vi "aggregator - pid.vi"(0 "df":dbl=100.0, 1 "low":dbl=1.0, 2 "threshold":dbl=1.0, 3 "dz":dbl=-9.0, 4 "dz0":dbl=-6.0, 5 "high":dbl=1.0, 6 "requested size":i32=10, 7 "P":dbl=0.1, 8 "negative":i32=2, 10 "first time":bool, 11 "I":dbl=1.0, 12 "requested averaging interval":i32=9, 13 "D":dbl=1.0) -> (14 "new df":dbl, 17 "above ?":bool, 18 "thershold ?":bool, 19 "heater":dbl)   [LabVIEW 2012]
panel:
  out "mean":dbl
  out "slope":dbl
  out "interpolated average":dbl
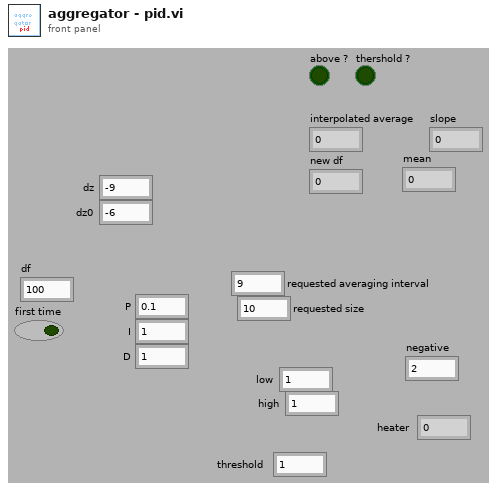
[diagram p1: front panel]
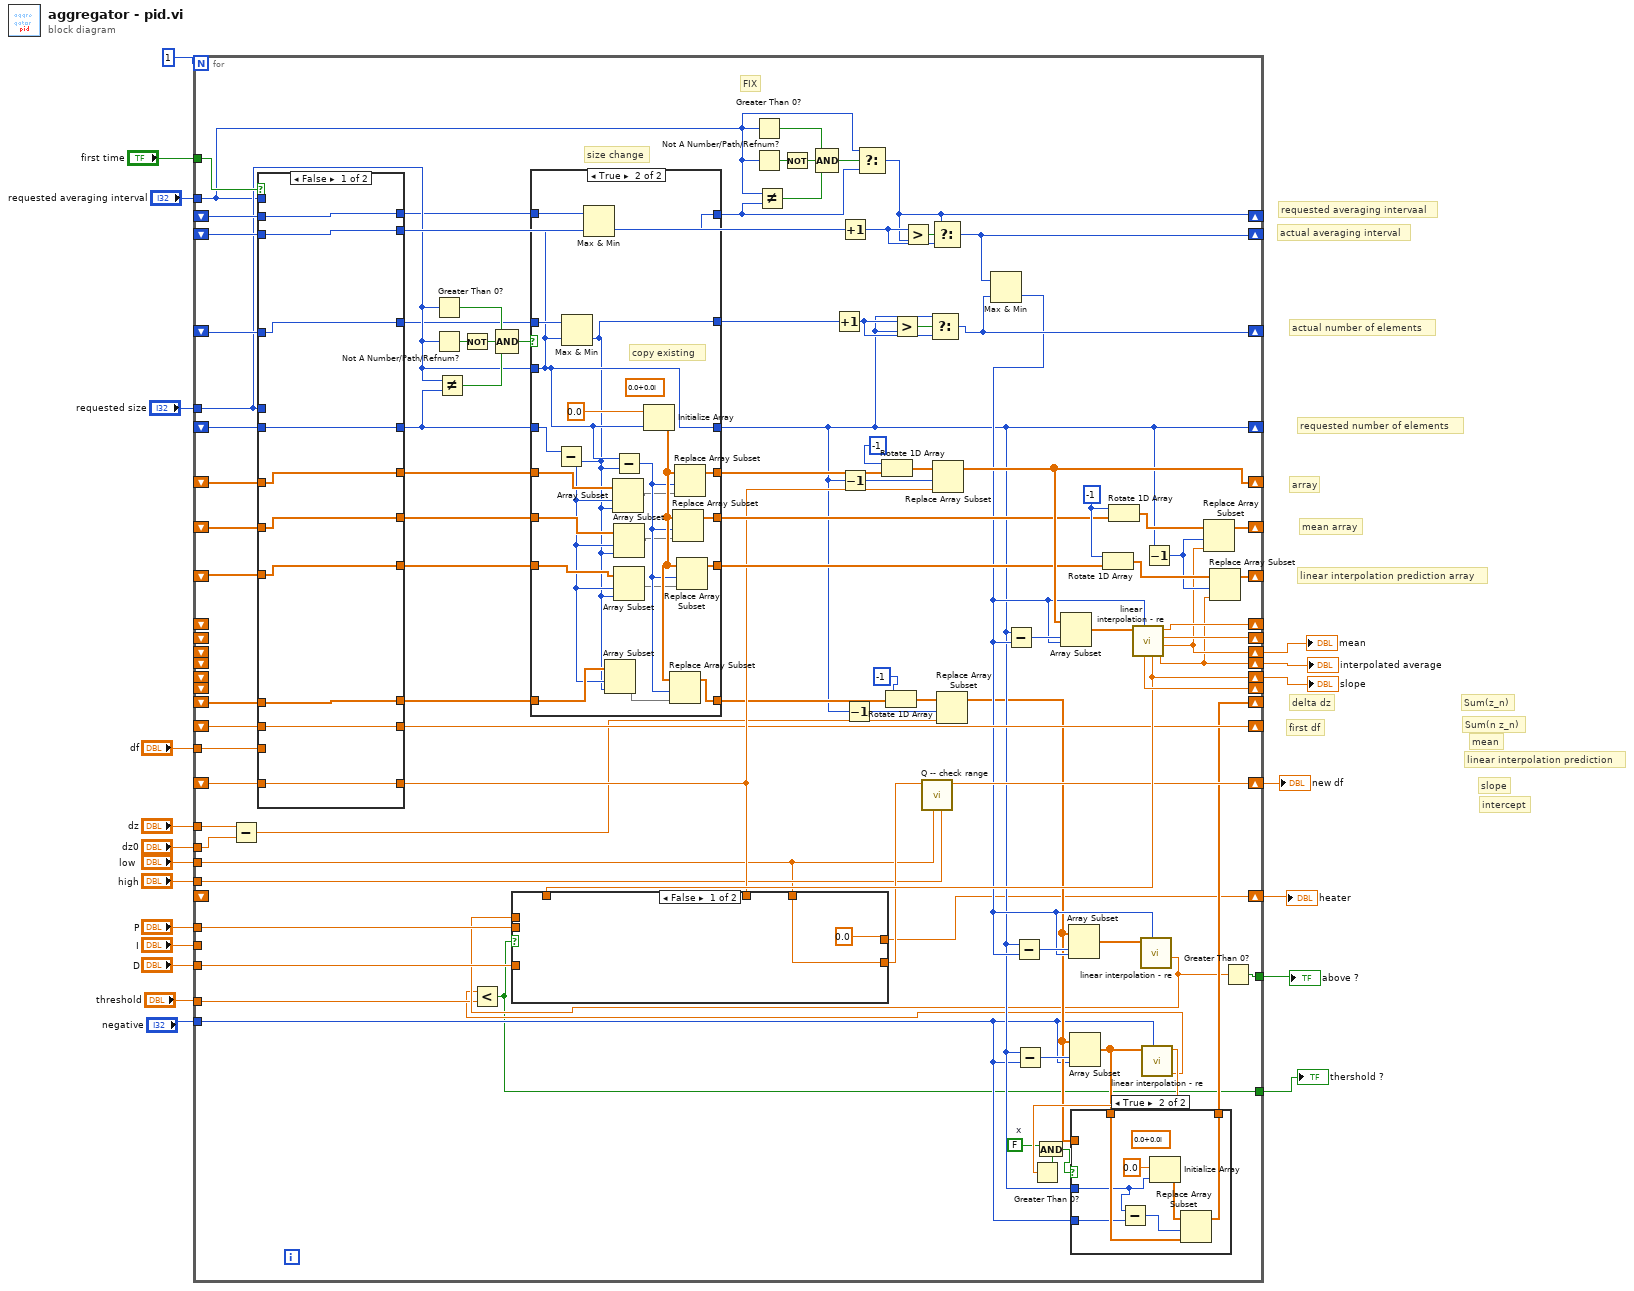
[diagram p0: block diagram]
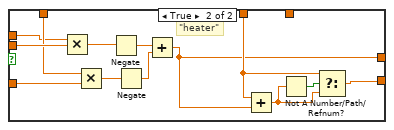
[diagram p2: hidden frame]
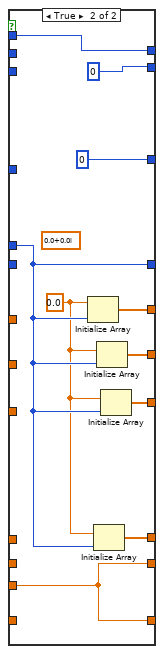
[diagram p5: hidden frame]
diagram:
  # "delta dz"
  # "first df"
  # "array"
  # "actual averaging interval"
  # "requested averaging intervaal"
  # "linear interpolation prediction"
  # "mean"
  # "intercept"
  # "slope"
  # "linear interpolation prediction array"
  # "mean array"
  # "Sum(n z_n)"
  # "Sum(z_n)"
  # "requested number of elements"
  # "actual number of elements"
  n1 = for {
    N: 1 -> [_]
    tunnel: "first time" -> [w94]
    shift-right: [w64] -> _
    shift-left: _ -> [w117]
    tunnel: "requested size" -> [w81]
    tunnel: "df" -> [w52]
    shift-right: [w96] -> _
    shift-left: _ -> [w114]
    shift-right: [w36] -> _
    shift-left: _ -> [w110]
    shift-right: [w103] -> _
    shift-left: _ -> [w109]
    shift-right: [w102] -> _
    shift-left: _ -> [w108]
    shift-right: [w92] -> _
    shift-left: _ -> [_]
    shift-right: [w91] -> _
    shift-left: _ -> [_]
    shift-right: [w57] -> w15
    shift-left: _ -> [_]
    shift-right: [w58] -> _
    shift-left: _ -> [_]
    shift-right: [w90] -> w14
    shift-left: _ -> [_]
    shift-right: [w89] -> w16
    shift-left: _ -> [_]
    shift-right: [w63] -> _
    shift-left: _ -> [w98]
    shift-right: [w65] -> _
    shift-left: _ -> [w97]
    tunnel: "requested averaging interval" -> [w67]
    tunnel: "P" -> [w62]
    tunnel: "dz" -> [w61]
    tunnel: "dz0" -> [w60]
    tunnel: "D" -> [w59]
    tunnel: "I" -> [_]
    shift-right: [w53] -> w8
    shift-left: _ -> [w55]
    shift-right: [w50] -> _
    shift-left: _ -> [w51]
    tunnel: "low" -> [w29]
    tunnel: "high" -> [w49]
    tunnel: [w48] -> w5
    shift-right: [w34] -> _
    shift-left: _ -> [w46]
    tunnel: "negative" -> [w32]
    shift-right: [w31] -> w3
    shift-left: _ -> [_]
    tunnel: "threshold" -> [w28]
    tunnel: [w22] -> w1
    w25 = FALSE  # x
    w105 = -1 ("n")
    # "FIX"
    # "size change"
    n2 = Subtract(x=w61, y=w60) -> (x-y=w24:dbl)
    n3 = case shown="False" w94 {
      tunnel: w117 -> [w178 _]
      tunnel: [w178 0] -> w79
      tunnel: w114 -> [w175 _]
      tunnel: w81 -> [_ w182]
      tunnel: w110 -> [w176 _]
      tunnel: w109 -> [w174 _]
      tunnel: w108 -> [w173 _]
      tunnel: [w175 w186] -> w83
      tunnel: [w174 w185] -> w76
      tunnel: [w173 w184] -> w77
      tunnel: [w179 0] -> w100
      tunnel: w98 -> [w179 _]
      tunnel: w67 -> [_ w187]
      tunnel: w97 -> [w177 _]
      tunnel: [w177 w187] -> w73
      tunnel: [w176 w182] -> w80
      tunnel: [w172 w183] -> w56
      tunnel: w52 -> [_ w183]
      tunnel: w55 -> [w172 _]
      tunnel: [w171 w183] -> w50
      tunnel: w51 -> [w171 _]
      tunnel: [w170 w180] -> w47
      tunnel: w46 -> [w170 _]
      frame False {
      }
      frame True {
        w181 = 0.0
        (unwired) cdb 0.0+0.0i
        n4 = Initialize Array(w181, w182) -> (w186:dbl[])
        n5 = Initialize Array(w181, w182) -> (w180:dbl[])
        n6 = Initialize Array(w181, w182) -> (w185:dbl[])
        n7 = Initialize Array(w181, w182) -> (w184:dbl[])
      }
    }
    n8 = Greater Than 0?(x=w81) -> (x > 0?=w87:bool)
    n9 = Not A Number/Path/Refnum?(number/path/refnum=w81) -> (NaN/Path/Refnum?=w88:bool)
    n10 = Not Equal?(x=w81, y=w80) -> (x != y?=w85:bool)
    n11 = Not(x=w88) -> (.not. x?=w86:bool)
    n12 = Compound Arithmetic op=AND(w87, w86, w85) -> (w84:bool)
    n13 = case shown="True" w84 {
      tunnel: [w147 w148] -> w78
      tunnel: w79 -> [w147 w169]
      tunnel: [w146 w163] -> w36
      tunnel: w80 -> [w146 w150]
      tunnel: [w145 w168] -> w82
      tunnel: w83 -> [w145 w154]
      tunnel: w81 -> [_ w163]
      tunnel: w77 -> [w143 w158]
      tunnel: w76 -> [w144 w156]
      tunnel: [w144 w167] -> w75
      tunnel: [w143 w166] -> w74
      tunnel: w73 -> [w142 w165]
      tunnel: [w142 w164] -> w66
      tunnel: w47 -> [w141 w152]
      tunnel: [w141 w159] -> w43
      frame False {
      }
      frame True {
        (unwired) cdb 0.0+0.0i
        # "copy existing"
        n14 = Max & Min(x=w169, y=w163) -> (min(x,y)=w148:i32)  [unwired: 1 out]
        n15 = Subtract(x=w150, y=w148) -> (x-y=w149:i32)
        n16 = Max & Min(x=w165, y=w163) -> (min(x,y)=w164:i32)  [unwired: 1 out]
        n17 = Array Subset(array=w152, index=w149, length=w148) -> (w151:dbl[])
        n18 = Array Subset(array=w154, index=w149, length=w148) -> (w153:dbl[])
        n19 = Subtract(x=w163, y=w148) -> (x-y=w160:i32)
        n20 = Array Subset(array=w156, index=w149, length=w148) -> (w155:dbl[])
        n21 = Array Subset(array=w158, index=w149, length=w148) -> (w157:dbl[])
        n22 = Initialize Array(0.0, w163) -> (w161:dbl[])
        n23 = Replace Array Subset(array=w161, new element=w151, index=w160) -> (w159:dbl[])
        n24 = Replace Array Subset(array=w161, new element=w155, index=w160) -> (w167:dbl[])
        n25 = Replace Array Subset(array=w161, new element=w153, index=w160) -> (w168:dbl[])
        n26 = Replace Array Subset(array=w161, new element=w157, index=w160) -> (w166:dbl[])
      }
    }
    n27 = Greater Than 0?(x=w67) -> (x > 0?=w71:bool)
    n28 = Not A Number/Path/Refnum?(number/path/refnum=w67) -> (NaN/Path/Refnum?=w72:bool)
    n29 = Not Equal?(x=w67, y=w66) -> (x != y?=w69:bool)
    n30 = Not(x=w72) -> (.not. x?=w70:bool)
    n31 = Compound Arithmetic op=AND(w71, w70, w69) -> (w68:bool)
    n32 = Increment(x=w78) -> (x+1=w115:i32)
    n33 = Increment(x=w100) -> (x+1=w99:i32)
    n34 = Decrement(x=w36) -> (x-1=w112:i32)
    n35 = Decrement(x=w36) -> (x-1=w45:i32)
    n36 = Select(t=w67, s=w68, f=w66) -> (s? t:f=w65:i32)
    n37 = Rotate 1D Array(1:w82, 2:-1 ("n")) -> (0:w111:dbl[])
    n38 = Rotate 1D Array(1:w43, 2:-1 ("n")) -> (0:w44:dbl[])
    n39 = Greater?(x=w115, y=w36) -> (0:w116:bool)
    n40 = Greater?(x=w99, y=w65) -> (0:w101:bool)
    n41 = Select(t=w36, s=w116, f=w115) -> (s? t:f=w64:i32)
    n42 = Select(t=w65, s=w101, f=w99) -> (s? t:f=w63:i32)
    n43 = Replace Array Subset(array=w111, new element=w56, index=w112) -> (w96:dbl[])
    n44 = Replace Array Subset(array=w44, new element=w24, index=w45) -> (w33:dbl[])
    n45 = Max & Min(x=w63, y=w64) -> (min(x,y)=w39:i32)  [unwired: 1 out]
    n46 = Subtract(x=w36, y=w39) -> (x-y=w95:i32)
    n47 = Subtract(x=w36, y=w39) -> (x-y=w41:i32)
    n48 = Subtract(x=w36, y=w32) -> (x-y=w38:i32)
    n49 = Array Subset(array=w96, index=w95, length=w39) -> (w93:dbl[])
    n50 = Array Subset(array=w33, index=w41, length=w39) -> (w40:dbl[])
    n51 = Array Subset(array=w33, index=w38, length=w32) -> (w35:dbl[])
    n52 = Rotate 1D Array(1:w74, 2:w105) -> (0:w106:dbl[])
    n53 = Rotate 1D Array(1:w75, 2:w105) -> (0:w107:dbl[])
    n54 = call "linear interpolation - re.vi"("n"=w39, "Array"=w93) -> ("interpolated average"=w89:dbl, "mean"=w90:dbl, "sum n z_n"=w91:dbl, "sum z_n"=w92:dbl, "slope"=w57:dbl, "intercept"=w58:dbl)  [unwired: 4 in]
    n55 = call "linear interpolation - re.vi"("n"=w39, "Array"=w40) -> ("mean"=w30:dbl)  [unwired: 4 in, 5 out]
    n56 = call "linear interpolation - re.vi"("n"=w32, "Array"=w35) -> ("interpolated average"=w23:dbl, "sum z_n"=w37:dbl)  [unwired: 4 in, 4 out]
    n57 = Less?(x=w23, y=w28) -> (x < y?=w22:bool)
    n58 = case shown="False" w22 {
      tunnel: w62 -> [_ w132]
      tunnel: w59 -> [_ w131]
      tunnel: w57 -> [_ w126]
      tunnel: w56 -> [_ w123]
      tunnel: [w119 w122] -> w54
      tunnel: [0.0 w121] -> w31
      tunnel: w30 -> [_ w120]
      tunnel: w29 -> [w119 _]
      frame False {
      }
      frame True {
        # "\"heater\""
        n59 = Multiply(x=w120, y=w132) -> (x*y=w130:dbl)
        n60 = Multiply(x=w126, y=w131) -> (x*y=w129:dbl)
        n61 = Negate(x=w130) -> (-x=w127:dbl)
        n62 = Negate(x=w129) -> (-x=w128:dbl)
        n63 = Add(x=w127, y=w128) -> (x+y=w121:dbl)
        n64 = Add(x=w123, y=w121) -> (x+y=w124:dbl)
        n65 = Not A Number/Path/Refnum?(number/path/refnum=w124) -> (NaN/Path/Refnum?=w125:bool)
        n66 = Select(t=w123, s=w125, f=w124) -> (s? t:f=w122:dbl)
      }
    }
    n67 = call "Q -- check range.vi"("upper"=w49, "lower"=w29, "number"=w54) -> ("number in range"=w53:dbl)  [unwired: 4 in, 4 out]
    n68 = Greater Than 0?(x=w37) -> (x > 0?=w26:bool)
    n69 = And(x=w25, y=w26) -> (x .and. y?=w27:bool)
    n70 = case shown="True" w27 {
      tunnel: w36 -> [_ w136]
      tunnel: w35 -> [_ w137]
      tunnel: w32 -> [_ w135]
      tunnel: [w133 w134] -> w34
      tunnel: w33 -> [w133 _]
      frame False {
      }
      frame True {
        (unwired) cdb 0.0+0.0i
        n71 = Subtract(x=w136, y=w135) -> (x-y=w138:i32)
        n72 = Initialize Array(0.0, w136) -> (w139:dbl[])
        n73 = Replace Array Subset(array=w139, new element=w137, index=w138) -> (w134:dbl[])
      }
    }
    n74 = Decrement(x=w36) -> (x-1=w104:i32)
    n75 = Replace Array Subset(array=w107, new element=w90, index=w104) -> (w103:dbl[])
    n76 = Replace Array Subset(array=w106, new element=w89, index=w104) -> (w102:dbl[])
    n77 = Greater Than 0?(x=w30) -> (x > 0?=w48:bool)
  }
  "interpolated average" <- w16
  "slope" <- w15
  "mean" <- w14
  "new df" <- w8
  "above ?" <- w5
  "heater" <- w3
  "thershold ?" <- w1
